vi "Read Float Configuration.vi"(7 "Type":T1, 8 "error in (no error)":errorcluster, 9 "Default If Not Found":ext=nan format="%#_17g", 10 "Name":string, 11 "IniFileSection in":refnum<class "IniFileSection.lvclass">) -> (0 "error out":errorcluster, 1 "Not Found?":bool, 2 "Value":ext format="%#_17g", 3 "IniFileSection out":refnum<class "IniFileSection.lvclass">)   [LabVIEW 2017, in "IniFileSection.lvclass"]
uses:
  IniFileSection.lvclass
  <vilib>/Utility/Data Type/Type Definitions/Data Type.ctl
  IniFileSection.lvclass/IniFileSection.ctl
  <vilib>/Utility/config.llb/NI_LVConfig.lvlib
  <vilib>/Utility/Data Type/NI_Data Type.lvlib
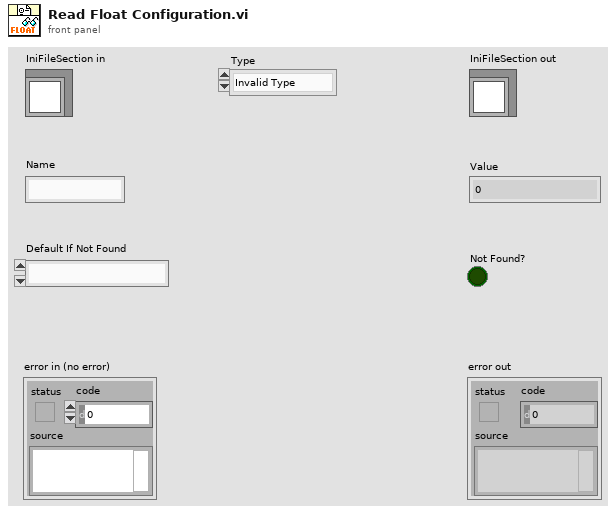
[diagram p1: front panel]
types:
  T1 = typedef "NI_Data Type.lvlib/Data Type.ctl" = enum8{"Invalid Type", "Void", "I8", "I16", "I32", "I64", "U8", "U16", "U32", "U64", "Single Float", "Double Float", "Extended Float", "Single Complex", "Double Complex", "Extended Complex", "Enum U8", "Enum U16", "Enum U32", "Enum U64", "Single Float With Unit", "Double Float With Unit", "Extended Float With Unit", "Single Complex with Unit", "Double Complex with Unit", "Extended Complex with Unit", "Boolean", "String", "Path", "Picture", "Tag", "Array", "Cluster", "Variant", "LV Variant", "Waveform", "Timestamp", "Digital Waveform", "Digital Data", "ExpressData", "Refnum", "External Data", "VI", "Poly VI", "LabVIEW Class Instance", "Fixed Point"}
  T2 = typedef "NI_LVConfig.lvlib/Config Data RefNum.ctl" = refnum<k1>
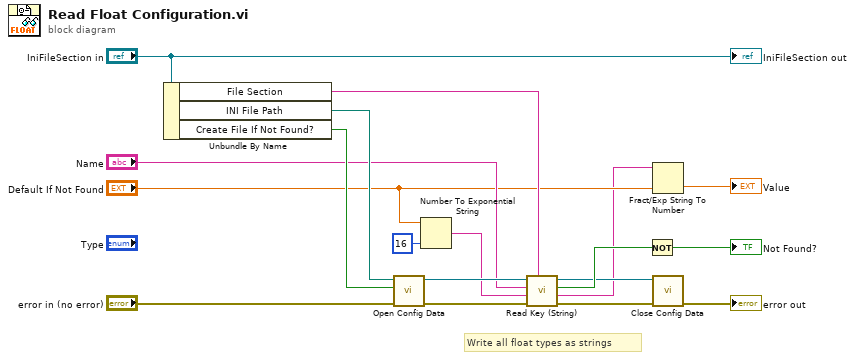
[diagram p0: block diagram]
diagram:
  # "Write all float types as strings"
  n1 = Unbundle By Name("IniFileSection in") -> ("File Section"=w7:string, "INI File Path"=w18:path, "Create File If Not Found?"=w14:bool)
  n2 = call <vilib>:"Open Config Data.vi"("error in (no error)"="error in (no error)", "create file if necessary (T)"=w14, "configuration file path"=w18) -> ("error out"=w12:errorcluster, "refnum"=w9:T2)  [unwired: 6 in, 1 out]
  n3 = Number To Exponential String(number="Default If Not Found", precision (6)=i16 16) -> (E-format string=w2:string)  [unwired: 2 in]
  n4 = call <vilib>:"Read Key (String).vi"("section"=w7, "error in (no error)"=w12, "default value"=w2, "key"="Name", "refnum"=w9) -> ("error out"=w11:errorcluster, "value"=w1:string, "found?"=w13:bool, "refnum out"=w10:T2)  [unwired: 3 in]
  n5 = Not(x=w13) -> (.not. x?=→"Not Found?":bool)
  n6 = Fract/Exp String To Number(string=w1, default (0 dbl)="Default If Not Found") -> (number=→"Value":ext)  [unwired: 2 in, 1 out]
  n7 = call <vilib>:"Close Config Data.vi"("error in (no error)"=w11, "refnum"=w10) -> ("error out"=→"error out":errorcluster)  [unwired: 8 in, 1 out]
  "IniFileSection out" <- "IniFileSection in"
